vi "Stop Core.vi"(10 "final error code":i32, 11 "UPNCalculator in":refnum<class "UPNCalculator.lvclass">) -> (3 "UPNCalculator out":refnum<class "UPNCalculator.lvclass">)   [LabVIEW 2016, in "UPNCalculator Actor.lvlib" / "UPNCalculator.lvclass"]
uses:
  UPNCalculator.lvclass
  <vilib>/ActorFramework/Time-Delayed Send Message/Time-Delay Override Options.ctl
  UPNCalculator.lvclass/UPNCalculator.ctl
  <vilib>/ActorFramework/Actor/Actor.lvclass
  Stack/Stack.lvclass
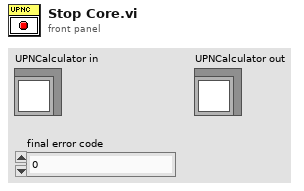
[diagram p1: front panel]
types:
  T1 = typedef "Time-Delay Override Options.ctl" = enum16{"Send next copy now", "Skip next scheduled copy", "Send next copy now and stop all further copies", "Stop all further copies"}
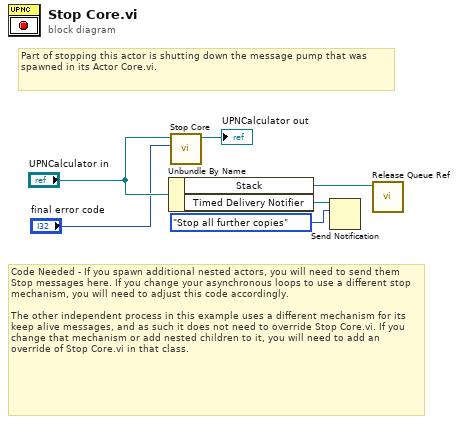
[diagram p0: block diagram]
diagram:
  # "Code Needed - If you spawn additional nested actors, you will need to send them Stop messages here. If you change your asynchronous loops to use a different stop mechanism, you will need to adjust this code accordingly.\n\nThe other independent process in this example uses a different mechanism for its keep alive messages, and as such it does not need to override Stop Core.vi. If you change that mechanism or add nested children to it, you will need to add an override of Stop Core.vi in that class."
  # "Part of stopping this actor is shutting down the message pump that was spawned in its Actor Core.vi."
  n1 = Unbundle By Name("UPNCalculator in") -> ("Stack"=w1:refnum<class "Stack.lvclass">, "Timed Delivery Notifier"=w4:refnum<notifier>)
  n2 = call-parent "Stop Core.vi"("final error code"="final error code", "Actor in"="UPNCalculator in") -> ("Actor out"=→"UPNCalculator out":refnum<class "UPNCalculator.lvclass">)  [unwired: 9 in]
  n3 = Send Notification(notification=Time-Delay_Override_Options."Stop all further copies", notifier=w4) -> ()  [unwired: 1 in, 2 out]
  n4 = call "Release Queue Ref.vi"("Stack in"=w1) -> ()  [unwired: 10 in, 1 out]
